vi "Format Data.vi"(2 "Error In":errorcluster, 4 "Indicators":T1) -> (0 "Error Out":errorcluster, 1 "Formatted Data String Out":string)   [LabVIEW 2020]
doc: "Format Data.vi takes the current iteration's Indicators Cluster as input and outputs a string that is formatted for the log file contained in the Record (save to Log Data File) subVI."
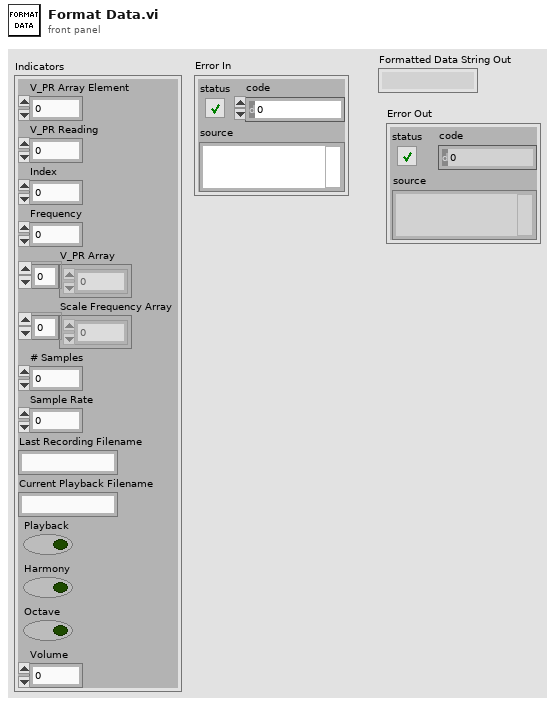
[diagram p1: front panel]
types:
  T1 = cluster{"V_PR Array Element":dbl, "V_PR Reading":dbl, "Index":i32, "Frequency":dbl, "V_PR Array":dbl[], "Scale Frequency Array":dbl[], "# Samples":i32, "Sample Rate":dbl, "Last Recording Filename":string, "Current Playback Filename":string, "Playback":bool, "Harmony":bool, "Octave":bool, "Volume":dbl}
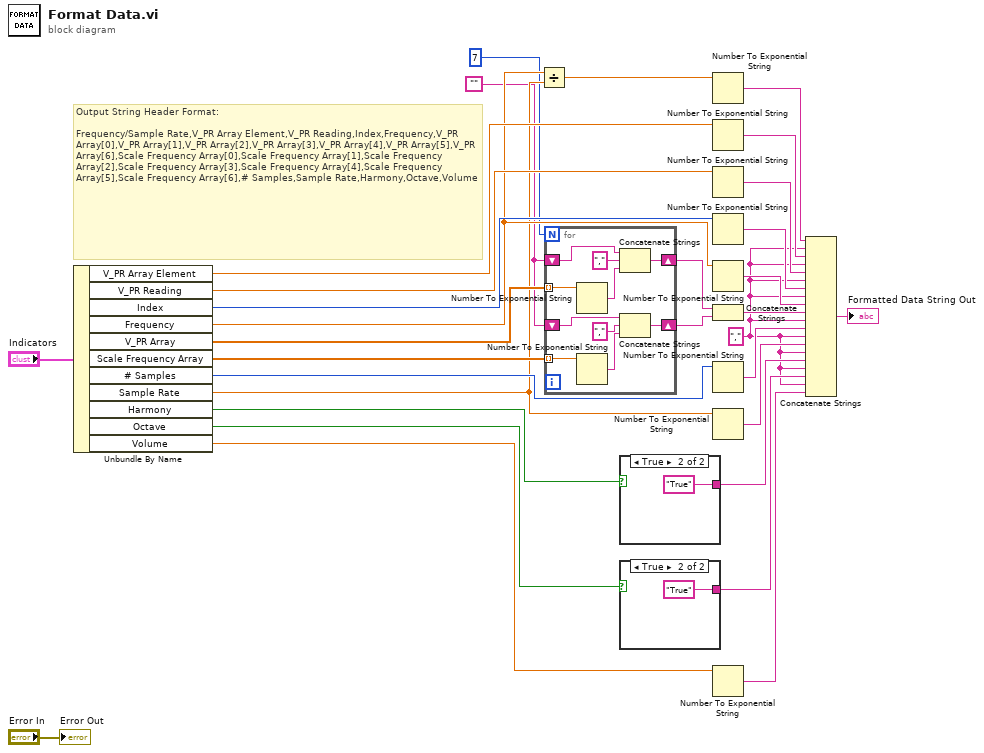
[diagram p0: block diagram]
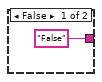
[diagram p2: hidden frame]
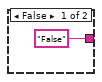
[diagram p3: hidden frame]
diagram:
  w7 = ""
  w9 = "," ("string")
  # "Output String Header Format:\n\nFrequency/Sample Rate,V_PR Array Element,V_PR Reading,Index,Frequency,V_PR Array[0],V_PR Array[1],V_PR Array[2],V_PR Array[3],V_PR Array[4],V_PR Array[5],V_PR Array[6],Scale Frequency Array[0],Scale Frequency Array[1],Scale Frequency Array[2],Scale Frequency Array[3],Scale Frequency Array[4],Scale Frequency Array[5],Scale Frequency Array[6],# Samples,Sample Rate,Harmony,Octave,Volume"
  n1 = Unbundle By Name("Indicators") -> ("V_PR Array Element"=w31:dbl, "V_PR Reading"=w27:dbl, "Index"=w25:i32, "Frequency"=w23:dbl, "V_PR Array"=w21:dbl[], "Scale Frequency Array"=w20:dbl[], "# Samples"=w16:i32, "Sample Rate"=w14:dbl, "Harmony"=w3:bool, "Octave"=w2:bool, "Volume"=w1:dbl)
  n2 = Divide(x=w23, y=w14) -> (x/y=w29:dbl)
  n3 = for {
    N: 7 -> [_]
    tunnel: w21 -> [w41] mode=indexing
    tunnel: w20 -> [w40] mode=indexing
    shift-right: [w37] -> w19
    shift-left: w7 -> [w36]
    shift-right: [w35] -> w18
    shift-left: w7 -> [w34]
    n4 = Number To Exponential String(number=w41) -> (E-format string=w38:string)  [unwired: 3 in]
    n5 = Number To Exponential String(number=w40) -> (E-format string=w32:string)  [unwired: 3 in]
    n6 = Concatenate Strings(w36, "," ("string"), w38) -> (w37:string)
    n7 = Concatenate Strings(w34, "," ("string"), w32) -> (w35:string)
  }
  n8 = case shown="True" w3 {
    tunnel: ["False" "True"] -> w11
    frame False {
    }
    frame True {
    }
  }
  n9 = case shown="True" w2 {
    tunnel: ["False" "True"] -> w10
    frame False {
    }
    frame True {
    }
  }
  n10 = Number To Exponential String(number=w29) -> (E-format string=w28:string)  [unwired: 3 in]
  n11 = Number To Exponential String(number=w31) -> (E-format string=w30:string)  [unwired: 3 in]
  n12 = Number To Exponential String(number=w27) -> (E-format string=w26:string)  [unwired: 3 in]
  n13 = Number To Exponential String(number=w25) -> (E-format string=w24:string)  [unwired: 3 in]
  n14 = Number To Exponential String(number=w23) -> (E-format string=w22:string)  [unwired: 3 in]
  n15 = Concatenate Strings(w19, w18) -> (w17:string)
  n16 = Number To Exponential String(number=w16) -> (E-format string=w15:string)  [unwired: 3 in]
  n17 = Number To Exponential String(number=w14) -> (E-format string=w13:string)  [unwired: 3 in]
  n18 = Number To Exponential String(number=w1) -> (E-format string=w8:string)  [unwired: 3 in]
  n19 = Concatenate Strings(w28, w9, w30, w9, w26, w9, w24, w9, w22, w17, w9, w15, w9, w13, w9, w11, w9, w10, w9, w8) -> (→"Formatted Data String Out":string)
  "Error Out" <- "Error In"
